vi "Construct.vi"(8 "error in":errorcluster, 11 "pxi slot":u8) -> (0 "error out":errorcluster, 3 "Shared Resources out":refnum<class "Shared Resources.lvclass">)   [LabVIEW 2020, in "AIM ARINC 429 Engine.lvlib" / "Implementation.lvlib" / "Shared Resources.lvclass"]
uses:
  Shared Resources.lvclass
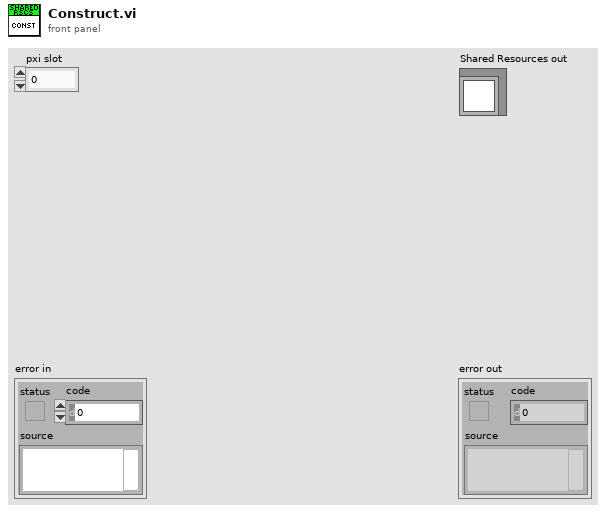
[diagram p1: front panel]
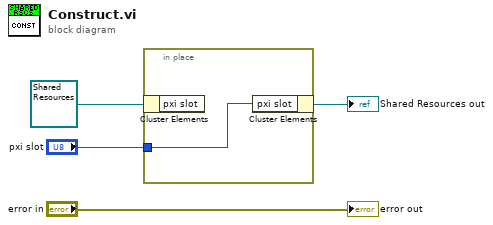
[diagram p0: block diagram]
diagram:
  n1 = in-place {
    in-place-border: "pxi slot" -> [w5]
    n2 = in-place-cluster #1(refnum<class "Shared Resources.lvclass"> refnum ("Communication Bus Template Interfaces:Implementation.lvlib:Shared Resources.lvclass")) -> ()  [unwired: 1 out]
    n3 = in-place-cluster #1("pxi slot"=w5) -> (→"Shared Resources out":refnum<class "Shared Resources.lvclass">)
  }
  "error out" <- "error in"
